vi "update.duration.vi"(8 "error in (no error)":errorcluster, 10 "Duration (s)":dbl, 11 "event in":refnum<class "event.lvclass">) -> (0 "error out":errorcluster, 3 "event out":refnum<class "event.lvclass">)   [LabVIEW 2020, in "event.lvclass"]
uses:
  event.lvclass
  event.lvclass/event.ctl
  Nominal Client/Nominal Client.lvclass
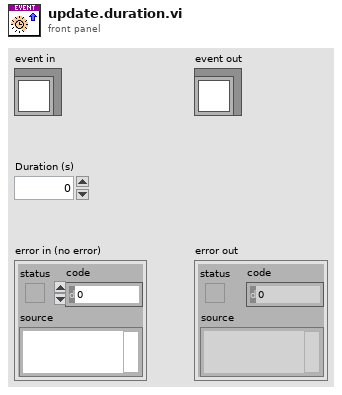
[diagram p1: front panel]
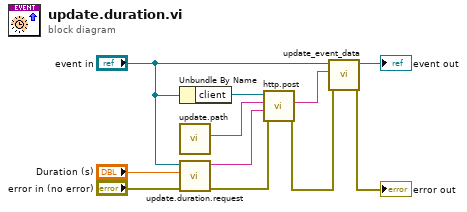
[diagram p0: block diagram]
diagram:
  n1 = Unbundle By Name("event in") -> ("client"=w11:refnum<class "Nominal Client.lvclass">)
  n2 = call "update.path.vi"() -> ("path"=w10:string)  [unwired: 11 in]
  n3 = call "update.duration.request.vi"("error in"="error in (no error)", "Duration (s)"="Duration (s)", "event"="event in") -> ("error out"=w9:errorcluster, "request"=w7:string)  [unwired: 7 in]
  n4 = call "http.post.vi"("error in"=w9, "Request body"=w7, "Path"=w10, "Nominal Client in"=w11) -> ("error out"=w3:errorcluster, "Response"=w6:string)  [unwired: 5 in, 1 out]
  n5 = call "update_event_data.vi"("error in"=w3, "JSON"=w6, "event in"="event in") -> ("error out"=→"error out":errorcluster, "event out"=→"event out":refnum<class "event.lvclass">)  [unwired: 7 in]
